vi "生成脉冲波形.vi"(8 "高速？":bool, 9 "limit I":dbl, 10 "脉宽":dbl, 11 "脉冲电压":string[][](array[string])) -> (3 "波形图":waveform(dbl))   [LabVIEW 2020, in "功能选择.xctl"]
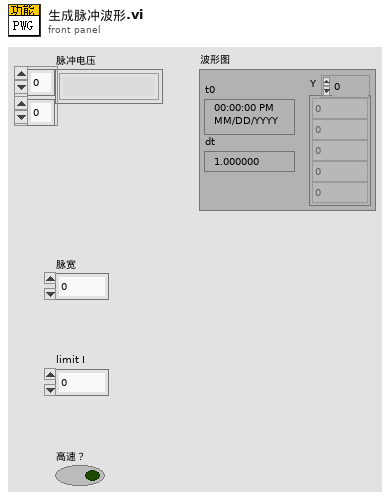
[diagram p1: front panel]
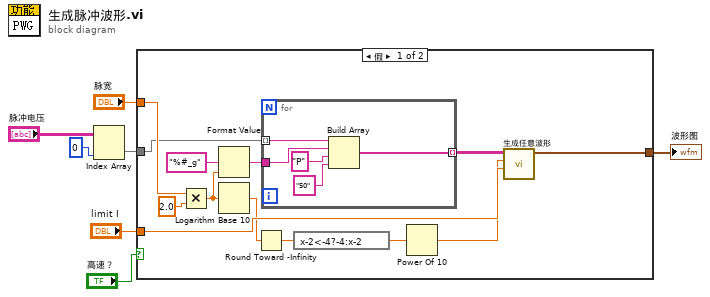
[diagram p0: block diagram]
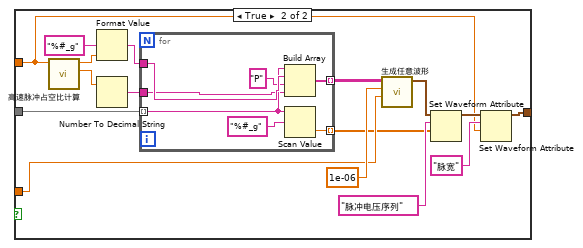
[diagram p2: hidden frame]
diagram:
  n1 = Index Array(array="脉冲电压", index (col)=0 ("禁用的索引 (列)")) -> (element=w1:string[])  [unwired: 1 in]
  n2 = case shown="假" "高速？" {
    tunnel: "脉宽" -> [w18 w33]
    tunnel: "limit I" -> [w17 w40]
    tunnel: [w16 w35] -> w6
    tunnel: w1 -> [w8 w32]
    frame False {
      n3 = Multiply(x=w18, y=2.0) -> (x*y=w12:dbl)
      n4 = Format Value(format string="%#_g" ("格式字符串"), value (0)=w12) -> (output string=w10:string)  [unwired: 1 in]
      n5 = Logarithm Base 10(1:w12) -> (0:w14:dbl)
      n6 = Round Toward -Infinity(1:w14) -> (0:w13:dbl)
      n7 = for {
        tunnel: w8 -> [w25] mode=indexing
        tunnel: w10 -> [w24]
        tunnel: [w21] -> w9 mode=indexing
        n8 = Build Array(w25, w24, "P" ("元素"), "50" ("元素")) -> (w21:string[])
      }
      n9 = expression code="x-2<-4?-4:x-2"(w13) -> (w15:dbl)
      n10 = Power Of 10(x=w15) -> (10^x=w11:dbl)
      n11 = call "生成任意波形.vi"("限流"=w17, "采样点"=w11, "波形描述"=w9) -> ("波形图"=w16:waveform(dbl))  [unwired: 8 in]
    }
    frame True {
      n12 = call "高速脉冲占空比计算.vi"("脉宽"=w33) -> ("占空比"=w27:dbl, "周期"=w38:dbl)  [unwired: 9 in]
      n13 = Format Value(format string="%#_g" ("格式字符串"), value (0)=w38) -> (output string=w30:string)  [unwired: 1 in]
      n14 = Number To Decimal String(number=w27) -> (decimal integer string=w26:string)  [unwired: 1 in]
      n15 = for {
        tunnel: w32 -> [w44] mode=indexing
        tunnel: w30 -> [w48]
        tunnel: [w46] -> w28 mode=indexing
        tunnel: [w43] -> w29 mode=indexing
        tunnel: w26 -> [w42]
        n16 = Build Array(w44, w48, "P" ("元素"), w42) -> (w46:string[])
        n17 = Scan Value(string=w44, format string="%#_g" ("格式字符串")) -> (value=w43:dbl)  [unwired: 1 in, 1 out]
      }
      n18 = call "生成任意波形.vi"("限流"=w40, "采样点"=1e-06, "波形描述"=w28) -> ("波形图"=w39:waveform(dbl))  [unwired: 8 in]
      n19 = Set Waveform Attribute(5:w29, 6:"脉冲电压序列" ("名称"), 7:w39) -> (3:w36:waveform(dbl))  [unwired: 1 in, 2 out]
      n20 = Set Waveform Attribute(5:w33, 6:"脉宽" ("名称"), 7:w36) -> (3:w35:waveform(dbl))  [unwired: 1 in, 2 out]
    }
  }
  "波形图" <- w6
